vi "RxPwr.vi"(0 "VISA IN":refnum<visa-resource-name>="GPIB1::16::INSTR", 3 "Measurement":string="InputRL", 4 "Channel":i32=1, 5 "error in":errorcluster, 7 "Measurement Parameter":string="B,1", 9 "Method":string="RPOWer", 11 "Receiver":string="POW", 13 "Cmd":string="*OPC?") -> (14 "VISA Out":refnum<visa-resource-name>="GPIB1::16::INSTR", 19 "error out":errorcluster)   [LabVIEW 2018]
uses:
  PNA-X.lvlib
panel:
  out "read buffer":string="+1\n"
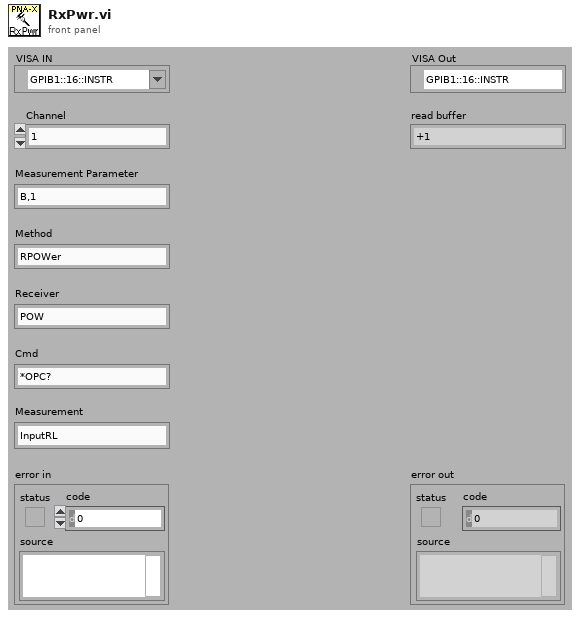
[diagram p1: front panel]
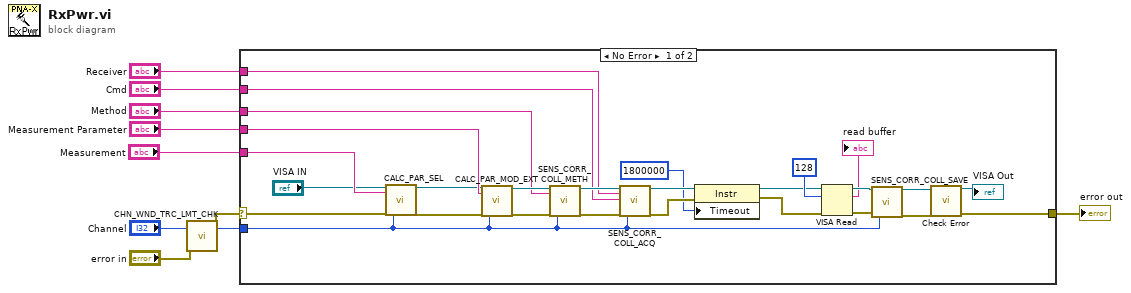
[diagram p0: block diagram]
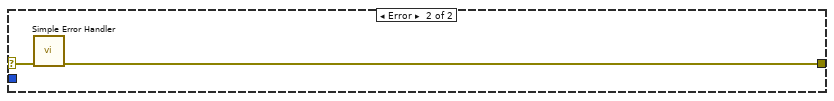
[diagram p2: hidden frame]
diagram:
  n1 = call "CHN_WND_TRC_LMT_CHK.vi"("Channel"="Channel", "error in"="error in") -> ("error out"=w3:errorcluster, "Channel"=w2:i32)  [unwired: 13 in, 3 out]
  n2 = case shown="No Error" w3 {
    selector: w3 -> [w22 w39]
    tunnel: [w37 w38] -> w9
    tunnel: "Measurement Parameter" -> [w29 _]
    tunnel: "Method" -> [w28 _]
    tunnel: "Cmd" -> [w27 _]
    tunnel: "Receiver" -> [w26 _]
    tunnel: w2 -> [w20 _]
    tunnel: "Measurement" -> [w19 _]
    frame No Error {
      n3 = call "CALC_PAR_SEL.vi"("VISA IN"="VISA IN", "Measurement"=w19, "error in"=w22, "Channel"=w20) -> ("VISA Out"=w21:refnum<visa-resource-name>, "error out"=w16:errorcluster)  [unwired: 14 in]
      n4 = call "CALC_PAR_MOD_EXT.vi"("VISA IN"=w21, "Measurement Parameter"=w29, "error in"=w16, "Channel"=w20) -> ("VISA Out"=w33:refnum<visa-resource-name>, "error out"=w35:errorcluster)  [unwired: 14 in]
      n5 = call "SENS_CORR_COLL_METH.vi"("VISA IN"=w33, "Method"=w28, "error in"=w35, "Channel"=w20) -> ("VISA Out"=w32:refnum<visa-resource-name>, "error out"=w34:errorcluster)  [unwired: 14 in]
      n6 = call "SENS_CORR_COLL_ACQ.vi"("VISA IN"=w32, "Reciever"=w26, "Cmd"=w27, "error in"=w34, "Channel"=w20) -> ("VISA Out"=w15:refnum<visa-resource-name>, "error out"=w14:errorcluster)  [unwired: 13 in]
      n7 = property class="Instr"(reference=w15, error in=w14, "Timeout"=1800000) -> (reference out=w12:refnum<visa-resource-name>, error out=w13:errorcluster)
      n8 = VISA Read(VISA resource name=w12, byte count=u32 128, error in (no error)=w13) -> (VISA resource name out=w25:refnum<visa-resource-name>, read buffer=→"read buffer":string, error out=w24:errorcluster)  [unwired: 1 out]
      n9 = call "SENS_CORR_COLL_SAVE.vi"("VISA IN"=w25, "error in"=w24, "Channel"=w20) -> ("VISA Out"=w30:refnum<visa-resource-name>, "error out"=w31:errorcluster)  [unwired: 15 in]
      n10 = call "Check Error.vi"("VISA Resource Name"=w30, "error in (no error)"=w31) -> ("dup VISA session"=→"VISA Out":refnum<visa-resource-name>, "error out"=w37:errorcluster)  [unwired: 16 in]
    }
    frame Error {
      n11 = call <vilib>:"Simple Error Handler.vi"("error in (no error)"=w39) -> ("error out"=w38:errorcluster)  [unwired: 4 in, 4 out]
    }
  }
  "error out" <- w9
